vi "PH_Sixpack.set i attribute.vi"(0 "i ref in":refnum<vi>, 2 "i attribute":T1={"Information"={"SixPack ID(0)"=0, "BaudRate(19200)"=19200, "COM Port"=enum."COM1", "HANDLE"=0}, "Serial Number"=-1.0, "Firmwareversion"=-1.0, "Axes"=[], "Status"=enum."None", "Axis to do a RefSearch"=-1, "GUI Refs"={"Information"=refnum, "Serial Number"=refnum, "Firmwareversion"=refnum, "Status"=refnum, "Axis to do a RefSearch"=refnum, "Axes Configuration (Sixpack)"=refnum, "Inputs"=refnum, "PeriodicInterval [ms]"=refnum}, "Constructor finished"=FALSE, "Ignore Error"=FALSE} {"Axes"."Config"."Axis Parameter"."Poslimit (6400)" step=1; "Axes"."Config"."Ref Search Parameter"."DebouncingTime (22ms)" format="%.0x"; "Axes"."Config"."I max (50%)" min=0.0 max=100.0}, 5 "error in (no error)":errorcluster) -> (14 "i ref out":refnum<vi>, 19 "error out":errorcluster)   [LabVIEW 2014, in "PH_Sixpack.lvlib"]
doc: "Sets the i attribute data of an object.\n\nLicense Agreement for this software:\n\nCopyright (C)\nGesellschaft für Schwerionenforschung, GSI\nPlanckstr. 1\n64291 Darmstadt\nGermany\n\nContact: D.Beck@gsi.de \n\nThis program is free software; you can redistribute it and/or modify it under the terms of the GNU General Public License as published by the Free Software Foundation; either version 2 of the license, or (at your option) any later version.\n\nThis program is distributed in the hope that it will be useful, but WITHOUT ANY WARRANTY; without even the implied warranty of MERCHANTABILITY or FITNESS FOR A PARTICULAR PURPOSE. See the GNU General License for more details (http://www.gnu.org).\n\nGesellschaft für Schwerionenforschung, GSI\nPlanckstr. 1, 64291 Darmstadt, Germany\nFor all questions and ideas contact: M.Richter@gsi.de, H.Brand@gsi.de or D.Beck@gsi.de.\nLast update: 17-JUN-2004"
uses:
  PH_Sixpack.lvlib
  PH_Sixpack.i attribute.ctl
  PH_Sixpack.Axis Cluster.ctl
  PH_Sixpack.Axis Configuration.ctl
  instr.lib/SixPack/PackDLL/VmaxAmax.ctl
  instr.lib/SixPack/PackDLL/PeakCurrent.ctl
  instr.lib/SixPack/PackDLL/VStartVmin.ctl
  instr.lib/SixPack/PackDLL/Ref Search Parameter.ctl
  instr.lib/SixPack/PackDLL/Stopswitch Limits.ctl
  instr.lib/SixPack/PackDLL/Motor Parameter.ctl
  instr.lib/SixPack/PackDLL/MotorParameter_P5.ctl
  instr.lib/SixPack/PackDLL/MotorParameter_P6.ctl
  instr.lib/SixPack/PackDLL/Current Control.ctl
  instr.lib/SixPack/PackDLL/Current.ctl
  PH_Sixpack.Status.ctl
  instr.lib/SixPack/Sixpack - Driver.lvlib
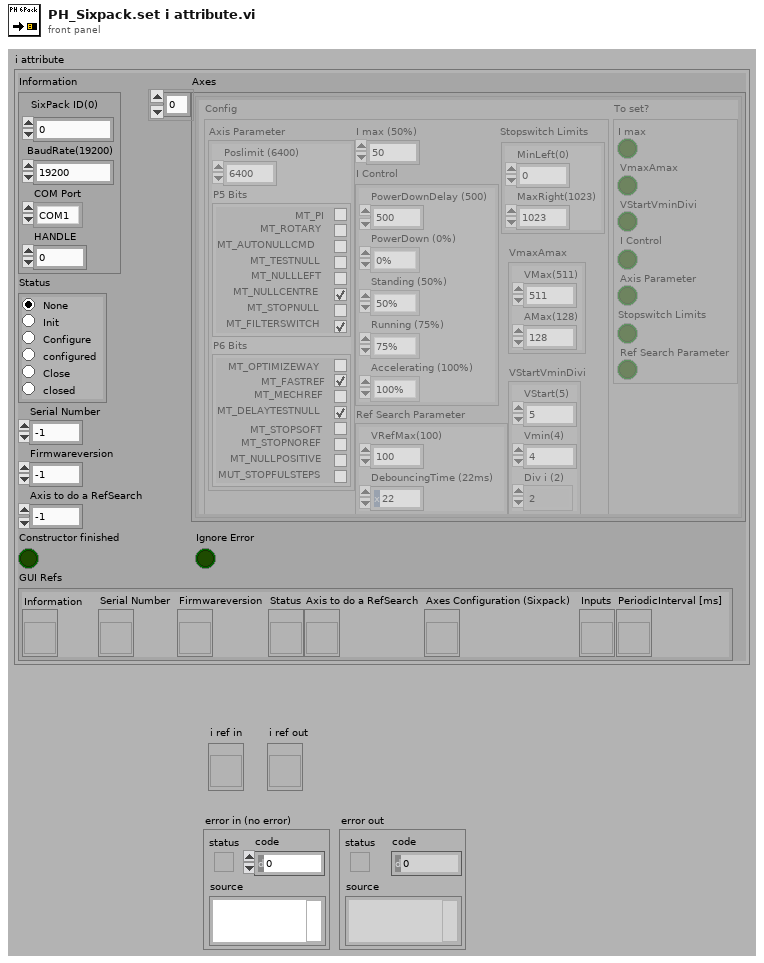
[diagram p1: front panel]
types:
  T1 = typedef "PH_Sixpack.lvlib/PH_Sixpack.i attribute.ctl" = cluster{"Information":cluster{"SixPack ID(0)":u16, "BaudRate(19200)":u16, "COM Port":enum32{"COM1", "COM2", "COM3", "COM4", "COM5", "COM6", "COM7", "COM8", "COM9"}, "HANDLE":i32}, "Serial Number":dbl, "Firmwareversion":dbl, "Axes":T2[], "Status":T14, "Axis to do a RefSearch":i32, "GUI Refs":cluster{"Information":refnum<vi>, "Serial Number":refnum<vi>, "Firmwareversion":refnum<vi>, "Status":refnum<vi>, "Axis to do a RefSearch":refnum<vi>, "Axes Configuration (Sixpack)":refnum<vi>, "Inputs":refnum<vi>, "PeriodicInterval [ms]":refnum<vi>}, "Constructor finished":bool, "Ignore Error":bool}
  T2 = typedef "PH_Sixpack.lvlib/PH_Sixpack.Axis Cluster.ctl" = cluster{"Config":T3, "To set?":cluster{"VmaxAmax":bool, "I max":bool, "VStartVminDivi":bool, "Ref Search Parameter":bool, "Stopswitch Limits":bool, "Axis Parameter":bool, "I Control":bool}}
  T3 = typedef "PH_Sixpack.lvlib/PH_Sixpack.Axis Configuration.ctl" = cluster{"VmaxAmax":T4, "I max (50%)":T5, "VStartVminDivi":T6, "Ref Search Parameter":T7, "Stopswitch Limits":T8, "Axis Parameter":T9, "I Control":T12}
  T4 = typedef "Sixpack - Driver.lvlib/VmaxAmax.ctl" = cluster{"VMax(511)":u16, "AMax(128)":u16}
  T5 = typedef "Sixpack - Driver.lvlib/PeakCurrent.ctl" = dbl
  T6 = typedef "Sixpack - Driver.lvlib/VStartVmin.ctl" = cluster{"VStart(5)":u16, "Vmin(4)":u16, "Div i (2)":enum8{"0", "1", "2", "3"}}
  T7 = typedef "Sixpack - Driver.lvlib/Ref Search Parameter.ctl" = cluster{"VRefMax(100)":u16, "DebouncingTime (22ms)":u8}
  T8 = typedef "Sixpack - Driver.lvlib/Stopswitch Limits.ctl" = cluster{"MinLeft(0)":u16, "MaxRight(1023)":u16}
  T9 = typedef "Sixpack - Driver.lvlib/Motor Parameter.ctl" = cluster{"Poslimit (6400)":u32, "P5 Bits":T10, "P6 Bits":T11}
  T10 = typedef "Sixpack - Driver.lvlib/MotorParameter_P5.ctl" = cluster{"MT_PI":bool, "MT_ROTARY":bool, "MT_AUTONULLCMD":bool, "MT_TESTNULL":bool, "MT_NULLLEFT":bool, "MT_NULLCENTRE":bool, "MT_STOPNULL":bool, "MT_FILTERSWITCH":bool}
  T11 = typedef "Sixpack - Driver.lvlib/MotorParameter_P6.ctl" = cluster{"MT_OPTIMIZEWAY":bool, "MT_FASTREF":bool, "MT_MECHREF":bool, "MT_DELAYTESTNULL":bool, "MT_STOPSOFT":bool, "MT_STOPNOREF":bool, "MT_NULLPOSITIVE":bool, "MUT_STOPFULSTEPS":bool}
  T12 = typedef "Sixpack - Driver.lvlib/Current Control.ctl" = cluster{"PowerDownDelay (500)":u16, "PowerDown (0%)":T13, "Standing (50%)":T13, "Running (75%)":T13, "Accelerating (100%)":T13}
  T13 = typedef "Sixpack - Driver.lvlib/Current.ctl" = enum8{"100%", "75%", "50%", "38%", "25%", "19%", "13%", "9%", "0%"}
  T14 = typedef "PH_Sixpack.lvlib/PH_Sixpack.Status.ctl" = enum32{"None", "Init", "Configure", "configured", "Close", "closed"}
  T15 = enum16{"SetAttribute", "GetAttribute", "CreateAttribute", "DestroyAttribute", "DestroyAllAtributes"}
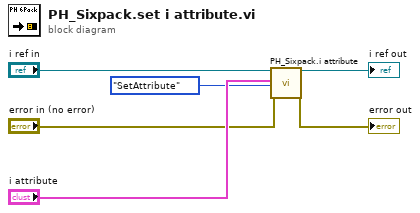
[diagram p0: block diagram]
diagram:
  n1 = call "PH_Sixpack.i attribute.vi"("VI Refnum"="i ref in", "CLASS.i attribute"="i attribute", "Action"=T15."SetAttribute", "error in (no error)"="error in (no error)") -> ("VI Refnum out"=→"i ref out":refnum<vi>, "error out"=→"error out":errorcluster)  [unwired: 13 in, 1 out]
